vi "Do.vi"(8 "error in (no error)":errorcluster, 10 "Actor in":refnum<class "Actor.lvclass">, 11 "Launch Model Msg":refnum<class "Launch Root Model Msg.lvclass">) -> (0 "error out":errorcluster, 2 "Actor out":refnum<class "Actor.lvclass">)   [LabVIEW 2015, in "IViewModel.lvlib" / "Launch Root Model Msg.lvclass"]
doc: "This VI delivers the message to the actor by calling the appropriate method(s) on the actor.\n\n<License>\nCopyright © 2017 Composed Systems, LLC | All rights reserved\nwww.composed.io\n\nAuthor: Ethan Stern <ethan.stern@composed.io>\n\nThis software is provided \"AS IS\" WITHOUT WARRANTIES, either express or implied, AND IS FOR EDUCATIONAL PURPOSES ONLY.\n</License>"
uses:
  Launch Root Model Msg.lvclass
  <vilib>/ActorFramework/Actor/Actor.lvclass
  IViewModel/IViewModel.lvclass
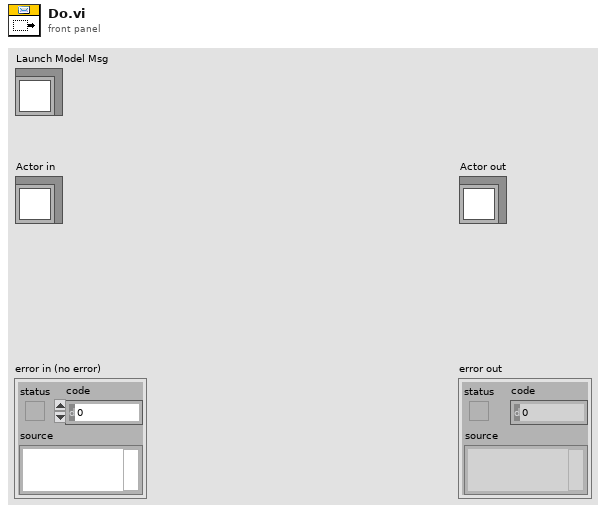
[diagram p1: front panel]
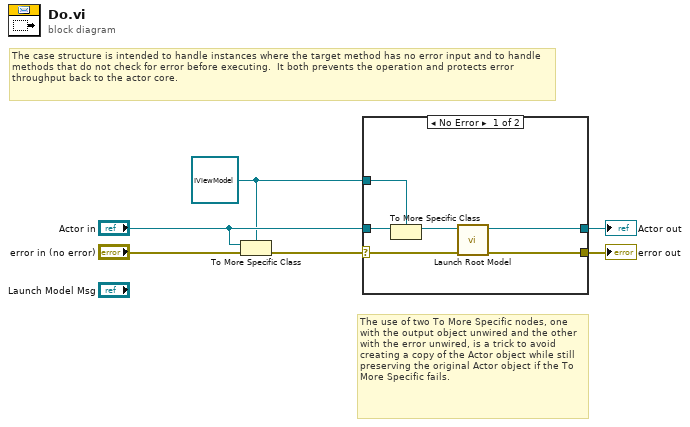
[diagram p0: block diagram]
diagram:
  w1 = refnum<class "IViewModel.lvclass"> refnum ("Actor in")
  # "The use of two To More Specific nodes, one with the output object unwired and the other with the error unwired, is a trick to avoid creating a copy of the Actor object while still preserving the original Actor object if the To More Specific fails."
  # "The case structure is intended to handle instances where the target method has no error input and to handle methods that do not check for error before executing.  It both prevents the operation and protects error throughput back to the actor core."
  n1 = To More Specific Class(target class=w1, reference="Actor in", error in="error in (no error)") -> (error out=w5:errorcluster)  [unwired: 1 out]
  n2 = case shown="No Error" w5 {
    selector: w5 -> [w10 w14]
    tunnel: [w12 w14] -> w4
    tunnel: [w11 w13] -> w3
    tunnel: "Actor in" -> [w9 w13]
    tunnel: w1 -> [w8 _]
    frame No Error {
      n3 = To More Specific Class(target class=w8, reference=w9) -> (specific class reference=w7:refnum<class "IViewModel.lvclass">)  [unwired: 1 in, 1 out]
      n4 = call-dynamic "Launch Root Model.vi"("error in (no error)"=w10, "IViewModel In"=w7) -> ("error out"=w12:errorcluster, "IViewModel Out"=w11:refnum<class "IViewModel.lvclass">)  [unwired: 8 in]
    }
    frame Error {
      # "If type check fails, pass the\noriginal object out again."
    }
  }
  "error out" <- w4
  "Actor out" <- w3
